vi "Test Process Multiple Stop.vi"(8 "error in (no error)":errorcluster, 11 "Process Test In":refnum<class "Process Test.lvclass">) -> (0 "error out":errorcluster, 3 "Process Test Out":refnum<class "Process Test.lvclass">)   [LabVIEW 2020, in "Process Test.lvclass"]
uses:
  Process Test.lvclass
  Framework/Process/Process.lvclass
  Mock Error Handler/Mock Error Handler.lvclass
  <vilib>/Asteme/LUnit/Test Case.lvclass
  C:/Users/anton/Documents/GitHub/Triarc-Framework/source/Framework/Process/Process.lvclass
  C:/Users/anton/Documents/GitHub/Triarc-Framework/source/Framework/Base/Base.lvclass
  C:/Users/anton/Documents/GitHub/Triarc-Framework/source/Framework/Configuration File/Configuration File.lvclass
  C:/Users/anton/Documents/GitHub/Triarc-Framework/source/Framework/Error Handler Interface/Error Handler Interface.lvclass
  C:/Users/anton/Documents/GitHub/Triarc-Framework/source/Framework Test/Mock Error Handler/Mock Error Handler.lvclass
  C:/Users/anton/Documents/GitHub/Triarc-Framework/source/Framework Test/Base Class Test/Base Test.lvclass
  C:/Program Files (x86)/National Instruments/LabVIEW 2020/vi.lib/Asteme/LUnit/Test Case.lvclass
  C:/Users/anton/Documents/GitHub/Triarc-Framework/source/Framework Test/Process Test/Process Test.lvclass
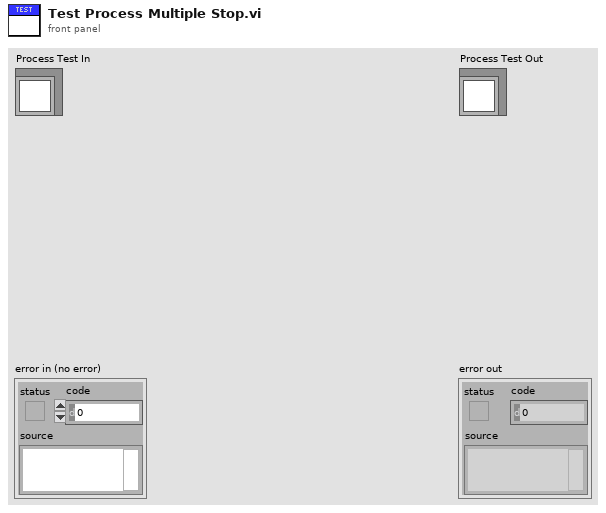
[diagram p1: front panel]
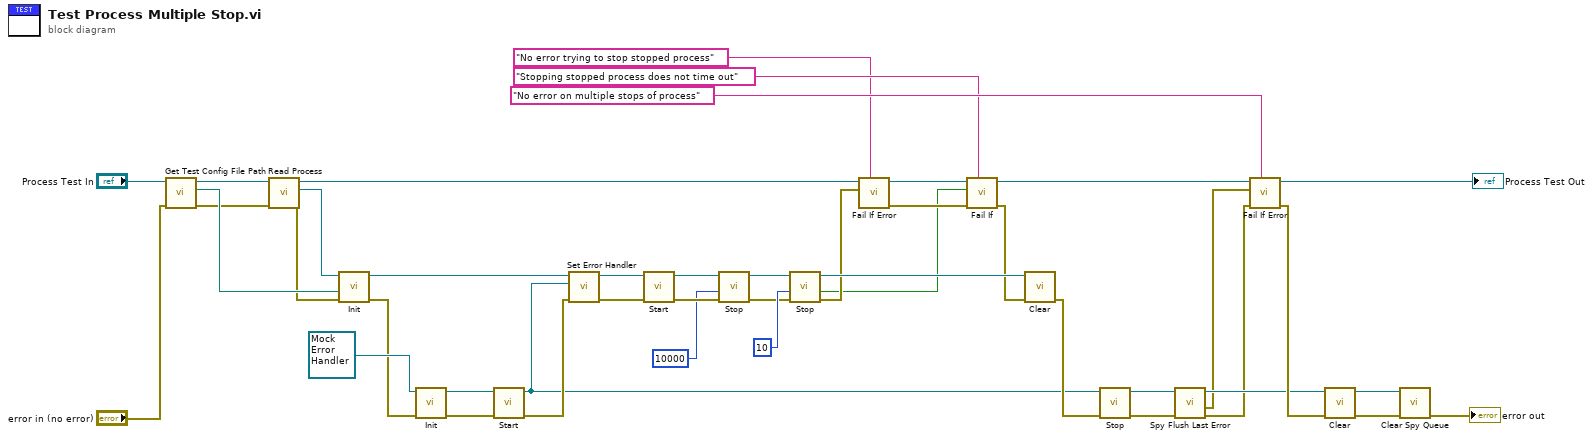
[diagram p0: block diagram]
diagram:
  n1 = call-dynamic "Get Test Config File Path.vi"("error in (no error)"="error in (no error)", "Base Class Test in"="Process Test In") -> ("error out"=w35:errorcluster, "Test config path"=w38:path, "Base Class Test out"=w40:refnum<class "Process Test.lvclass">)  [unwired: 7 in]
  n2 = call "Read Process.vi"("error in (no error)"=w35, "Process Test in"=w40) -> ("error out"=w36:errorcluster, "Process.lvclass"=w37:refnum<class "Process.lvclass">, "Process Test out"=w10:refnum<class "Process Test.lvclass">)  [unwired: 7 in]
  n3 = call-dynamic "Init.vi"("error in (no error)"=w36, "Config File Path"=w38, "Process In"=w37) -> ("error out"=w26:errorcluster, "Process Out"=w41:refnum<class "Process.lvclass">)  [unwired: 7 in]
  n4 = call-dynamic "Init.vi"("error in (no error)"=w26, "Mock Error Handler In"=refnum<class "Mock Error Handler.lvclass"> refnum ("Mock Error Handler.lvclass")) -> ("error out"=w30:errorcluster, "Mock Error Handler Out"=w29:refnum<class "Mock Error Handler.lvclass">)  [unwired: 8 in]
  n5 = call "Start.vi"("error in (no error)"=w30, "Process In"=w29) -> ("error out"=w25:errorcluster, "Process Out"=w17:refnum<class "Mock Error Handler.lvclass">)  [unwired: 8 in]
  n6 = call "Set Error Handler.vi"("error in (no error)"=w25, "Error Handler"=w17, "Process In"=w41) -> ("error out"=w31:errorcluster, "Process Out"=w32:refnum<class "Process.lvclass">)  [unwired: 7 in]
  n7 = call "Start.vi"("error in (no error)"=w31, "Process In"=w32) -> ("error out"=w43:errorcluster, "Process Out"=w44:refnum<class "Process.lvclass">)  [unwired: 8 in]
  n8 = call "Stop.vi"("error in (no error)"=w43, "timeout in ms (-1)"=10000, "Process In"=w44) -> ("error out"=w6:errorcluster, "Process Out"=w34:refnum<class "Process.lvclass">)  [unwired: 6 in, 1 out]
  n9 = call "Stop.vi"("error in (no error)"=w6, "timeout in ms (-1)"=10, "Process In"=w34) -> ("error out"=w5:errorcluster, "timed out?"=w3:bool, "Process Out"=w33:refnum<class "Process.lvclass">)  [unwired: 6 in]
  n10 = call <vilib>:"Fail If Error.vi"("Description"="No error trying to stop stopped process", "Assert error"=w5, "Test Case In"=w10) -> ("error out"=w13:errorcluster, "Test Case Out"=w14:refnum<class "Process Test.lvclass">)  [unwired: 7 in]
  n11 = call <vilib>:"Fail If.vi"("Description"="Stopping stopped process does not time out", "error in (no error)"=w13, "Fail?"=w3, "Test Case In"=w14) -> ("error out"=w4:errorcluster, "Test Case Out"=w9:refnum<class "Process Test.lvclass">)  [unwired: 6 in]
  n12 = call-dynamic "Clear.vi"("error in (no error)"=w4, "Process In"=w33) -> ("error out"=w24:errorcluster)  [unwired: 8 in, 1 out]
  n13 = call "Stop.vi"("error in (no error)"=w24, "Process In"=w17) -> ("error out"=w22:errorcluster, "Process Out"=w18:refnum<class "Mock Error Handler.lvclass">)  [unwired: 7 in, 1 out]
  n14 = call "Spy Flush Last Error.vi"("error in (no error)"=w22, "Mock Error Handler In"=w18) -> ("error out"=w2:errorcluster, "Errors"=w1:errorcluster, "Mock Error Handler Out"=w21:refnum<class "Mock Error Handler.lvclass">)  [unwired: 6 in, 1 out]
  n15 = call <vilib>:"Fail If Error.vi"("Description"="No error on multiple stops of process", "error in (no error)"=w2, "Assert error"=w1, "Test Case In"=w9) -> ("error out"=w23:errorcluster, "Test Case Out"=→"Process Test Out":refnum<class "Process Test.lvclass">)  [unwired: 6 in]
  n16 = call-dynamic "Clear.vi"("error in (no error)"=w23, "Process In"=w21) -> ("error out"=w19:errorcluster, "Process Out"=w20:refnum<class "Mock Error Handler.lvclass">)  [unwired: 8 in]
  n17 = call-dynamic "Clear Spy Queue.vi"("error in (no error)"=w19, "Mock Process In"=w20) -> ("error out"=→"error out":errorcluster)  [unwired: 8 in, 1 out]
